vi "PathPlanner_Cmd_FollowRamsetePathPack.vi"(8 "ControlPastEnd_Sec":dbl=3.0, 9 "Trigger Events":bool=TRUE, 10 "ReplanningConfig":T1={"enableInitialReplanning"=TRUE, "enableDynamicReplanning"=FALSE, "dynamicReplanningTotalErrorThreshold"=1.0, "dynamicReplanningErrorSpikeThreshold"=0.25}, 11 "RAMSETE_EXE_TUNING":T2={"B"=2.0, "Zeta"=0.7, "X Tolerance M"=2.0, "Y Tolerance M"=0.7, "Heading Tolerance RAD"=0.7, "Track Width M"=2.0, "Max Speed M/S"=2.0} {"Max Speed M/S" format="%13.4f"; "Track Width M" format="%13.4f"; "Heading Tolerance RAD" format="%13.4f"; "Y Tolerance M" format="%13.4f"; "X Tolerance M" format="%13.4f"; "Zeta" format="%13.4f"; "B" format="%13.4f"}) -> (3 "PathPlanner_Ctrl_RamDrvConfig":T3={"ControlPastEnd_Sec"=3.0, "ReplanningConfig"={"enableInitialReplanning"=TRUE, "enableDynamicReplanning"=FALSE, "dynamicReplanningTotalErrorThreshold"=1.0, "dynamicReplanningErrorSpikeThreshold"=0.25}, "Trigger Events"=TRUE, "RAMSETE_EXE_TUNING SI"={"B"=2.0, "Zeta"=0.7, "X Tolerance M"=2.0, "Y Tolerance M"=0.7, "Heading Tolerance RAD"=0.7, "Track Width M"=2.0, "Max Speed M/S"=2.0}} {"RAMSETE_EXE_TUNING SI"."Max Speed M/S" format="%13.4f"; "RAMSETE_EXE_TUNING SI"."Track Width M" format="%13.4f"; "RAMSETE_EXE_TUNING SI"."Heading Tolerance RAD" format="%13.4f"; "RAMSETE_EXE_TUNING SI"."Y Tolerance M" format="%13.4f"; "RAMSETE_EXE_TUNING SI"."X Tolerance M" format="%13.4f"; "RAMSETE_EXE_TUNING SI"."Zeta" format="%13.4f"; "RAMSETE_EXE_TUNING SI"."B" format="%13.4f"})   [LabVIEW 2019, in "PathPlanner24.lvlib"]
doc: "Pack controller tuning configuration for Path Planner Holonomic Drive Controller.\n\nInputs:\n - X PID Tuning - cluster - Input from PACK PROF PID VI\n - Y PID Tuning - cluster - Input from PACK PROF PID VI\n - thetaController - cluster - A profiled PID controller to respond to error in angle.\n - Max Wheel Speed M/.S - double - Maximum wheel speed (M/S)\n - DriveBaseRadius - double - The radius of the drive base in meters. For swerve drive, this is the\n distance from the center of the robot to the furthest module. For \n mecanum, this is the drive base width / 2\n - X Tolerance - double - X tolerance for calculating At Reference (Meters) (Optional. Default: 0.0762 )\n - Y Tolerance - double - Y tolerance for calculating At Reference (Meters) (Optional. Default: 0.0762 )\n - Rotation Tolerance - double - Rotation tolerance for calculating At Reference (Degrees) (Optional. Default: 0.0)873)\n\nOutputs:\n -- PathPlannerHolCtrlConfig -- cluster - packed controller configuration."
uses:
  PathPlanner24.lvlib
  TypeDef/PathPlannerCmdFollowRamConfig.ctl
  TypeDef/PathPlannerReplanningConfig.ctl
  <vilib>/Rock Robotics/WPI/ThirdParty/JAS_Junk/TrajLib/TypeDef/RAMSETE_EXE_TUNING.ctl
  <vilib>/Rock Robotics/WPI/ThirdParty/JAS_Junk/TrajLib/Rotation2d_CreateAngle.vi
  <vilib>/Rock Robotics/WPI/ThirdParty/JAS_Junk/TrajLib/Translation2d_Create.vi
  <vilib>/Rock Robotics/WPI/ThirdParty/JAS_Junk/TrajLib/Trajectory_Library.lvlib
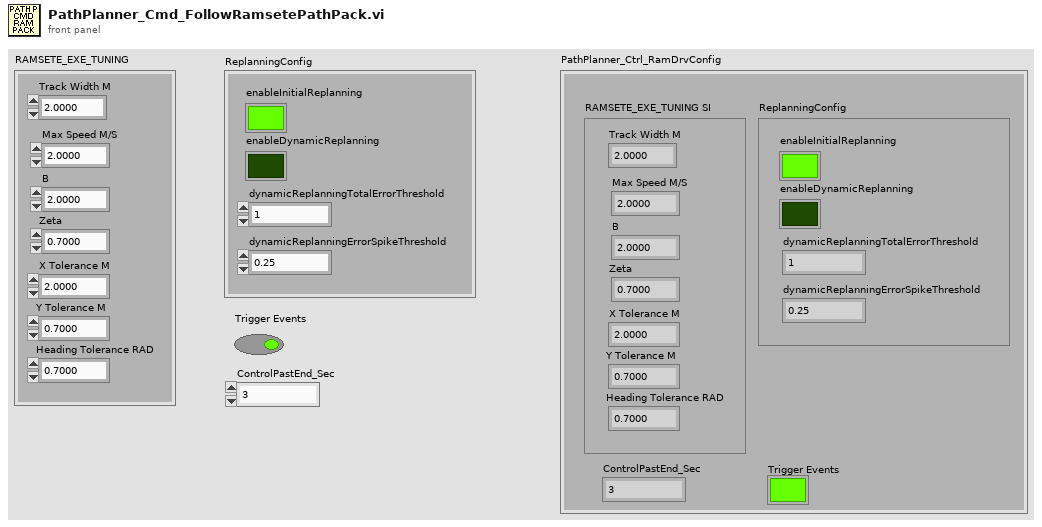
[diagram p1: front panel]
types:
  T1 = typedef "PathPlanner24.lvlib/PathPlannerReplanningConfig.ctl" = cluster{"enableInitialReplanning":bool, "enableDynamicReplanning":bool, "dynamicReplanningTotalErrorThreshold":dbl, "dynamicReplanningErrorSpikeThreshold":dbl}
  T2 = typedef "Trajectory_Library.lvlib/RAMSETE_EXE_TUNING.ctl" = cluster{"B":dbl, "Zeta":dbl, "X Tolerance M":dbl, "Y Tolerance M":dbl, "Heading Tolerance RAD":dbl, "Track Width M":dbl, "Max Speed M/S":dbl}
  T3 = typedef "PathPlanner24.lvlib/PathPlannerCmdFollowRamConfig.ctl" = cluster{"ControlPastEnd_Sec":dbl, "ReplanningConfig":T1, "Trigger Events":bool, "RAMSETE_EXE_TUNING SI":T2}
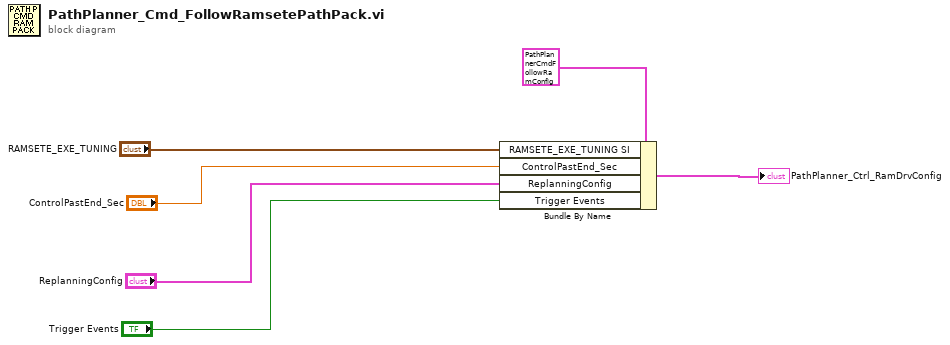
[diagram p0: block diagram]
diagram:
  n1 = Bundle By Name(cluster=T3 {"ControlPastEnd_Sec"=3.0, "ReplanningConfig"={"enableInitialReplanning"=TRUE, "enableDynamicReplanning"=FALSE, "dynamicReplanningTotalErrorThreshold"=1.0, "dynamicReplanningErrorSpikeThreshold"=0.25}, "Trigger Events"=TRUE, "RAMSETE_EXE_TUNING SI"={"B"=2.0, "Zeta"=0.7, "X Tolerance M"=2.0, "Y Tolerance M"=0.7, "Heading Tolerance RAD"=0.7, "Track Width M"=2.0, "Max Speed M/S"=2.0}} ("PathPlanner_Cmd_FollowRamConfig"), "RAMSETE_EXE_TUNING SI"="RAMSETE_EXE_TUNING", "ControlPastEnd_Sec"="ControlPastEnd_Sec", "ReplanningConfig"="ReplanningConfig", "Trigger Events"="Trigger Events") -> (→"PathPlanner_Ctrl_RamDrvConfig":T3)
